vi "例程31-基本混合单频VI的使用.vi"() -> ()   [LabVIEW 2016]
uses:
  <vilib>/measure/NI_MAPro.lvlib
panel:
  out "波形图":waveform(dbl)(graph)
  out "error out":errorcluster caption="错误输出"
  out "actual tone frequencies":dbl[](array[numeric]) caption="实际单频信号频率"
  out "crest factor":dbl caption="峰值因数" format="%.2p"
  out "signal out":waveform(dbl) caption="信号输出"
  in  "phase relationship":u16(ring) caption="相位关系" items=["随机", "线性差", "线性相位"]
  in  "coerce frequencies?":bool caption="强制转换频率？"
  in  "sampling info":cluster{"Fs":dbl, "#s":dbl}={"Fs"=1000.0, "#s"=1000.0} caption="采样信息" {"Fs" format="%.2p"}
  in  "error in (no error)":errorcluster caption="错误输入（无错误）"
  in  "delta frequency":dbl=100.0 caption="delta频率" format="%.2p"
  in  "seed":i32=-1 caption="种子"
  in  "amplitude":dbl=-1.0 caption="幅值" format="%.2p"
  in  "reset signal":bool caption="重置信号"
  in  "#tones":i32=3 caption="单频个数"
  in  "start frequency":dbl=10.0 caption="起始频率" format="%.2p"
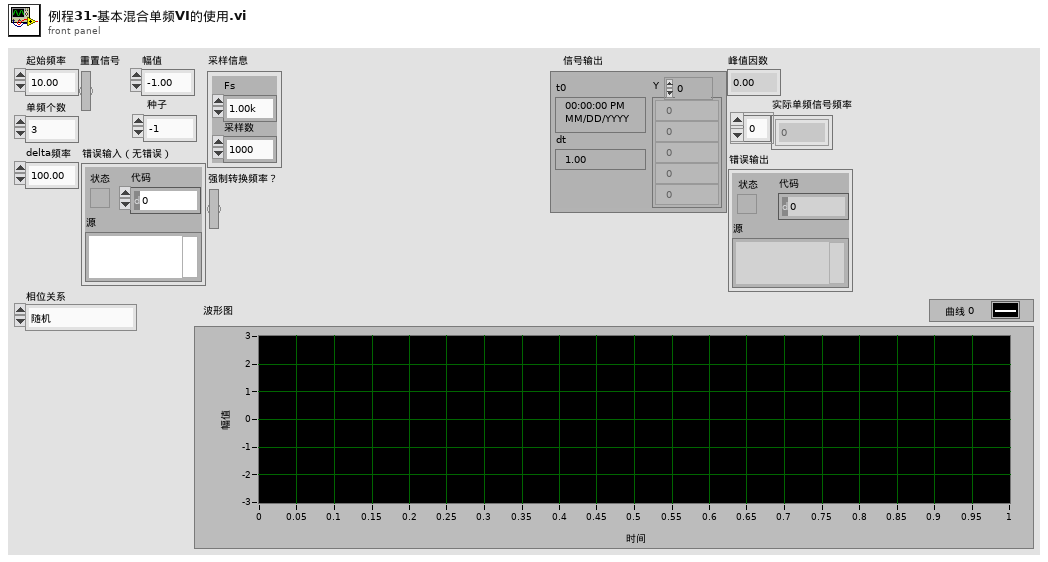
[diagram p1: front panel]
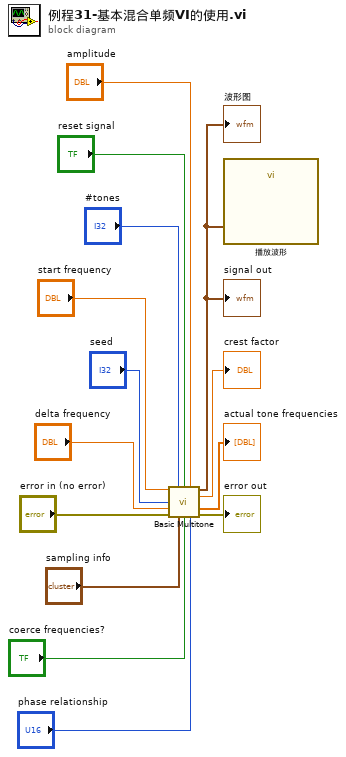
[diagram p0: block diagram]
diagram:
  n1 = call <vilib>:"Basic Multitone.vi"("start frequency"="start frequency", "#tones"="#tones", "reset signal"="reset signal", "amplitude"="amplitude", "seed"="seed", "delta frequency"="delta frequency", "error in (no error)"="error in (no error)", "sampling info"="sampling info", "coerce frequencies?"="coerce frequencies?", "phase relationship"="phase relationship") -> ("signal out"=w1:waveform(dbl), "crest factor"=→"crest factor":dbl, "actual tone frequencies"=→"actual tone frequencies":dbl[], "error out"=→"error out":errorcluster)  [unwired: 2 in]
  "signal out" <- w1
  "波形图" <- w1
  n2 = call "播放波形"("Data"=w1) -> ()  [unwired: 18 in, 1 out]
